vi "StartTimerSubVI.vi"(11 "Wait Time (Seconds)":dbl=4.0) -> (3 "End Time (Seconds)":dbl)   [LabVIEW 2019, in "Chapter2-Ex1-Library.lvlib"]
uses:
  Chapter2-Ex1-Library.lvlib
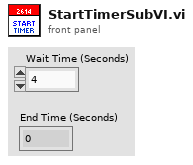
[diagram p1: front panel]
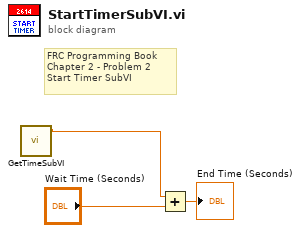
[diagram p0: block diagram]
diagram:
  # "FRC Programming Book\nChapter 2 - Problem 2\nStart Timer SubVI"
  n1 = call "GetTimeSubVI.vi"() -> ("Seconds"=w1:dbl)  [unwired: 11 in]
  n2 = Add(x=w1, y="Wait Time (Seconds)") -> (x+y=→"End Time (Seconds)":dbl)
